vi "Test Begin 2.vi"() -> ()   [LabVIEW 2014, in "Arduino SoftwareSerial Wrapper.lvlib"]
uses:
  Arduino SoftwareSerial Wrapper.lvlib
panel:
  out "Error Out":errorcluster
  in  "Error In":errorcluster
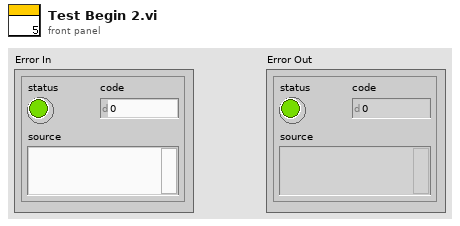
[diagram p1: front panel]
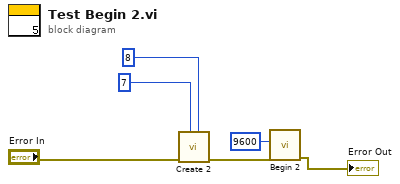
[diagram p0: block diagram]
diagram:
  n1 = call "Create 2.vi"("arduino RX pin"=u8 8 ("RX pin"), "arduino TX pin"=u8 7 ("RX pin"), "Error In"="Error In") -> ("Error Out"=w3:errorcluster)  [unwired: 8 in]
  n2 = call "Begin 2.vi"("Error In"=w3, "Baudrate"=u16 9600) -> ("Error Out"=→"Error Out":errorcluster)  [unwired: 8 in]
